vi "Launch.vi"(8 "error in (no error)":errorcluster, 10 "JQMHStartup":refnum<class "RQMHStartup.lvclass">, 11 "JQMHCore in":refnum<class "RQMHModule.lvclass">) -> (0 "error out":errorcluster)   [LabVIEW 2024, in "RQMHModule.lvclass"]
uses:
  RQMHModule.lvclass
  Startup/RQMHStartup.lvclass
  ModuleSD.vi
  RQMHModule.lvclass/RQMHModule.ctl
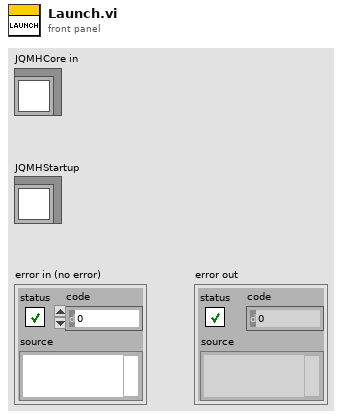
[diagram p1: front panel]
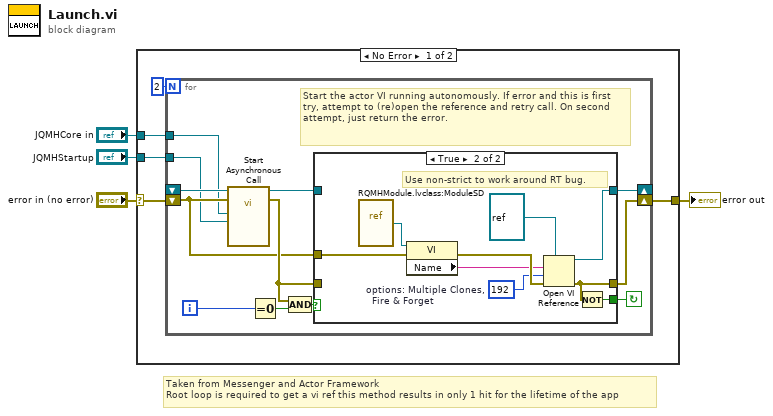
[diagram p0: block diagram]
diagram:
  # "Taken from Messenger and Actor Framework\nRoot loop is required to get a vi ref this method results in only 1 hit for the lifetime of the app"
  n1 = case shown="No Error" "error in (no error)" {
    selector: "error in (no error)" -> [w7 w33]
    tunnel: [w8 w33] -> w2
    tunnel: "JQMHCore in" -> [w6 _]
    tunnel: "JQMHStartup" -> [w5 _]
    frame No Error {
      n2 = for {
        N: 2 -> [_]
        shift-right: [w21] -> _
        shift-left: _ -> [w20]
        shift-right: [w18] -> w8
        shift-left: w7 -> [w12]
        tunnel: w6 -> [w11]
        tunnel: w5 -> [w10]
        i -> [w15]
        stop <- w13 continue-if-true
        # "Start the actor VI running autonomously. If error and this is first try, attempt to (re)open the reference and retry call. On second attempt, just return the error."
        n3 = call-by-ref "Start Asynchronous Call"(reference=w20, error in=w12, "JQMHStartup.lvclass"=w10, "JQMHCore in"=w11) -> (reference out=w19:refnum<vi>, error out=w14:errorcluster)  [unwired: 10 in]
        n4 = Equal To 0?(x=w15) -> (x = 0?=w16:bool)
        n5 = Compound Arithmetic op=AND(w14, w16) -> (w17:bool)
        n6 = case shown="True" w17 {
          tunnel: [w23 w29] -> w21
          tunnel: [w22 w27] -> w18
          tunnel: w19 -> [w23 _]
          tunnel: w14 -> [w22 _]
          tunnel: [_ w28] -> w13
          tunnel: w12 -> [_ w26]
          frame False {
          }
          frame True {
            w30 = 192  # options: Multiple Clones,   Fire & Forget
            # "Use non-strict to work around RT bug."
            n7 = vi-ref "RQMHModule.lvclass:ModuleSD.vi"() -> (w25:refnum<vi>)
            n8 = property class="VI"(reference=w25, error in=w26) -> (error out=w32:errorcluster, "Name"=w31:string)  [unwired: 1 out]
            n9 = Open VI Reference(type specifier VI Refnum (for type only)=refnum<vi> refnum, vi path=w31, options=w30, error in (no error)=w32) -> (vi reference=w29:refnum<vi>, error out=w27:errorcluster)  [unwired: 2 in]
            n10 = Not(x=w27) -> (.not. x?=w28:bool)
          }
        }
      }
    }
    frame Error {
    }
  }
  "error out" <- w2
